vi "V2analysis.vi"(0 "node_in":T2, 1 "VIPathMap":map{string, bool}(c390), 2 "GObj引用句柄":refnum<vi>, 3 "additional_params":T1, 4 "集合":set{string}(c389)) -> (7 "node_out":T2, 8 "VIPathMap 2":map{string, bool}(c390), 10 "集合 2":set{string}(c389))   [LabVIEW 2020]
uses:
  node.ctl
  terminalData.ctl
  terminal_type.ctl
  terminal_direction.ctl
  additional_params.ctl
panel:
  out "依赖关系:丢失依赖关系名称":string[](array[string])
  out "result string":string
  # "tunnel/judge/shift?"
  # "tunnel/judge/shift?"
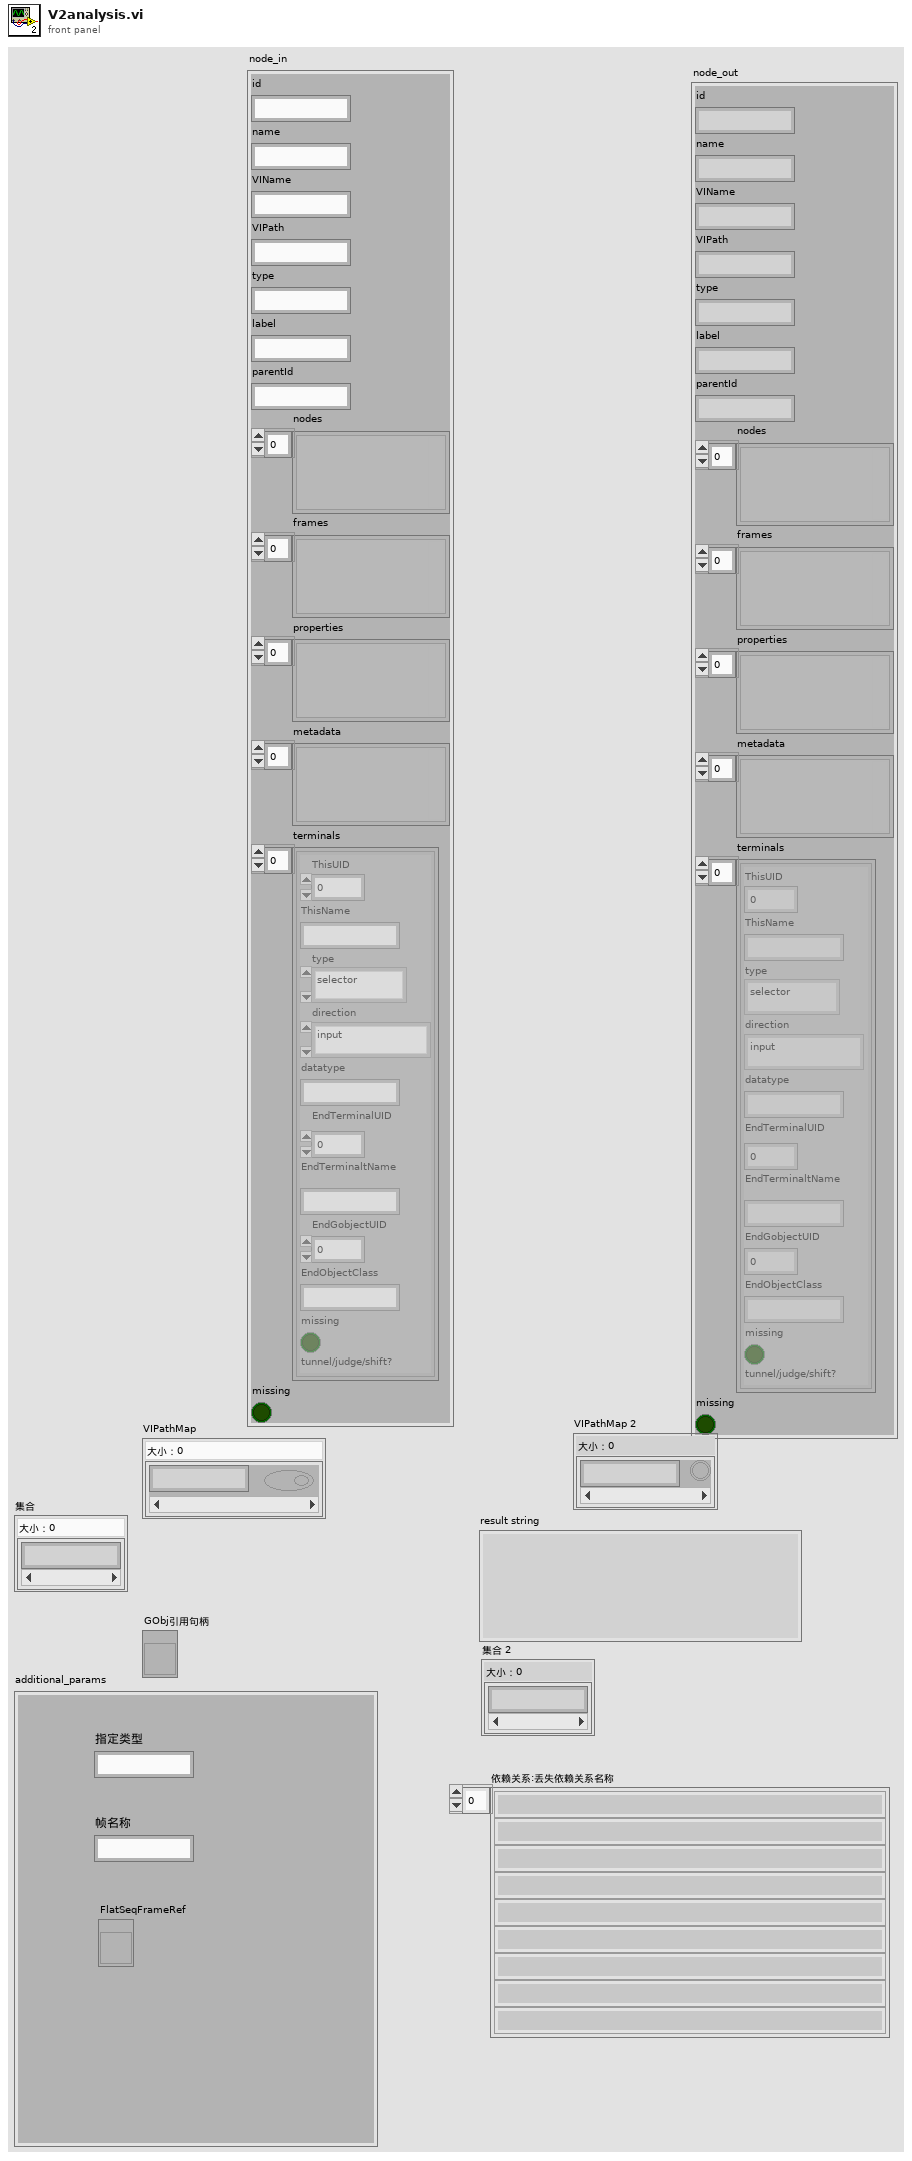
[diagram p1: front panel]
types:
  T1 = typedef "additional_params.ctl" = cluster{"指定类型":string, "帧名称":string, "FlatSeqFrameRef":refnum<vi>}
  T2 = typedef "node.ctl" = cluster{"id":string, "name":string, "VIName":string, "VIPath":string, "type":string, "label":string, "parentId":string, "nodes":variant[], "frames":variant[], "properties":variant[], "metadata":variant[], "terminals":T3[], "missing":bool}
  T3 = typedef "terminalData.ctl" = cluster{"ThisUID":i32, "ThisName":string, "type":T4, "direction":T5, "datatype":string, "EndTerminalUID":i32, "EndTerminaltName":string, "EndGobjectUID":i32, "EndObjectClass":string, "missing":bool}
  T4 = typedef "terminal_type.ctl" = enum16{"selector", "tunnel", "shift", "timeout", "normal", "floating"}
  T5 = typedef "terminal_direction.ctl" = enum16{"input", "output"}
  T6 = cluster{"casename":string, "subdia_text":string}[]
  T7 = cluster{"seq_name":string, "subdia_text":string}[]
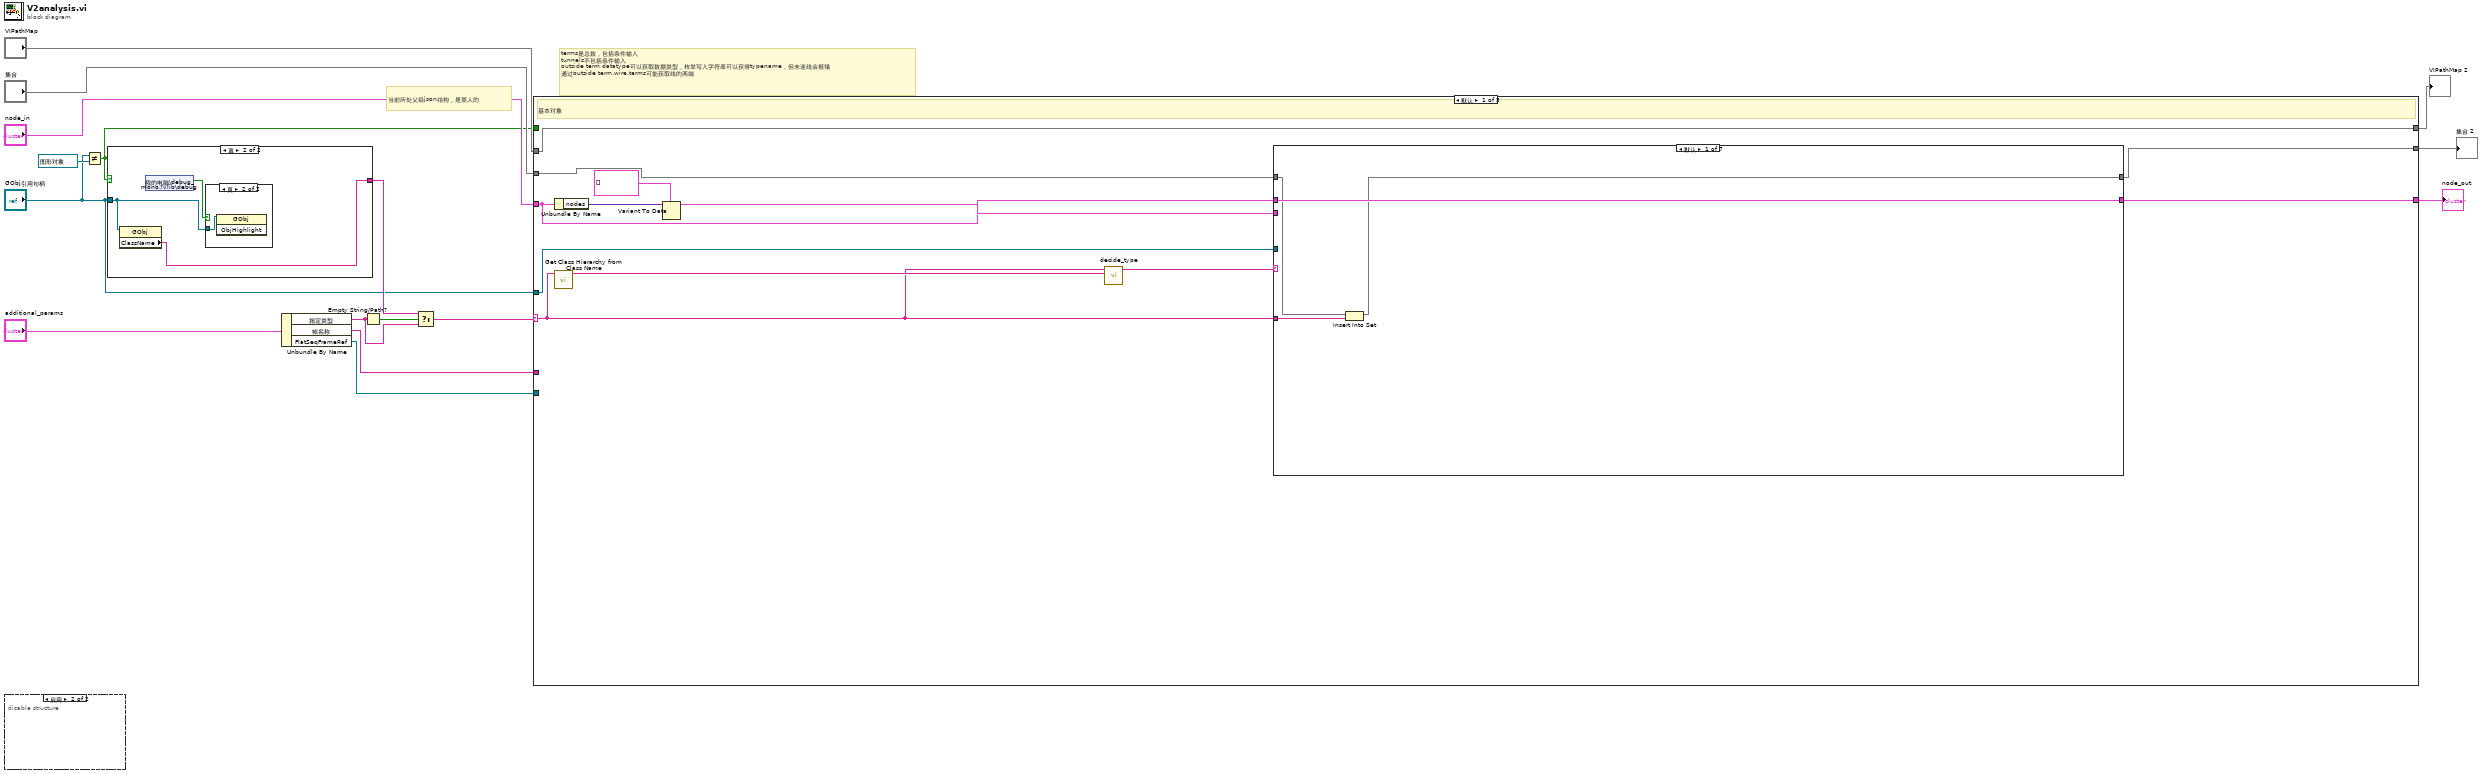
[diagram p0: block diagram]
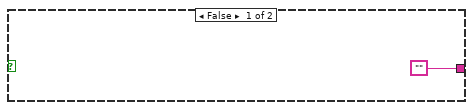
[diagram p2: hidden frame]
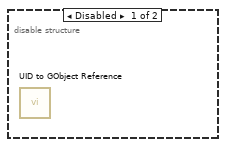
[diagram p4: hidden frame]
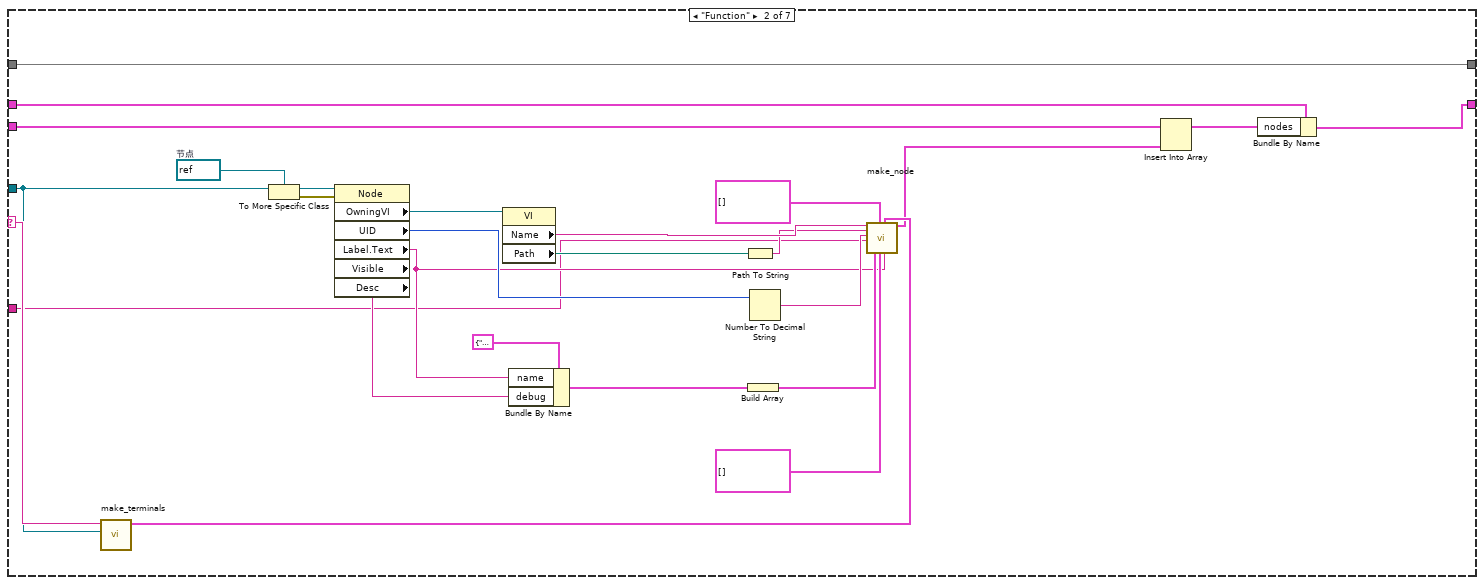
[diagram p5: hidden frame]
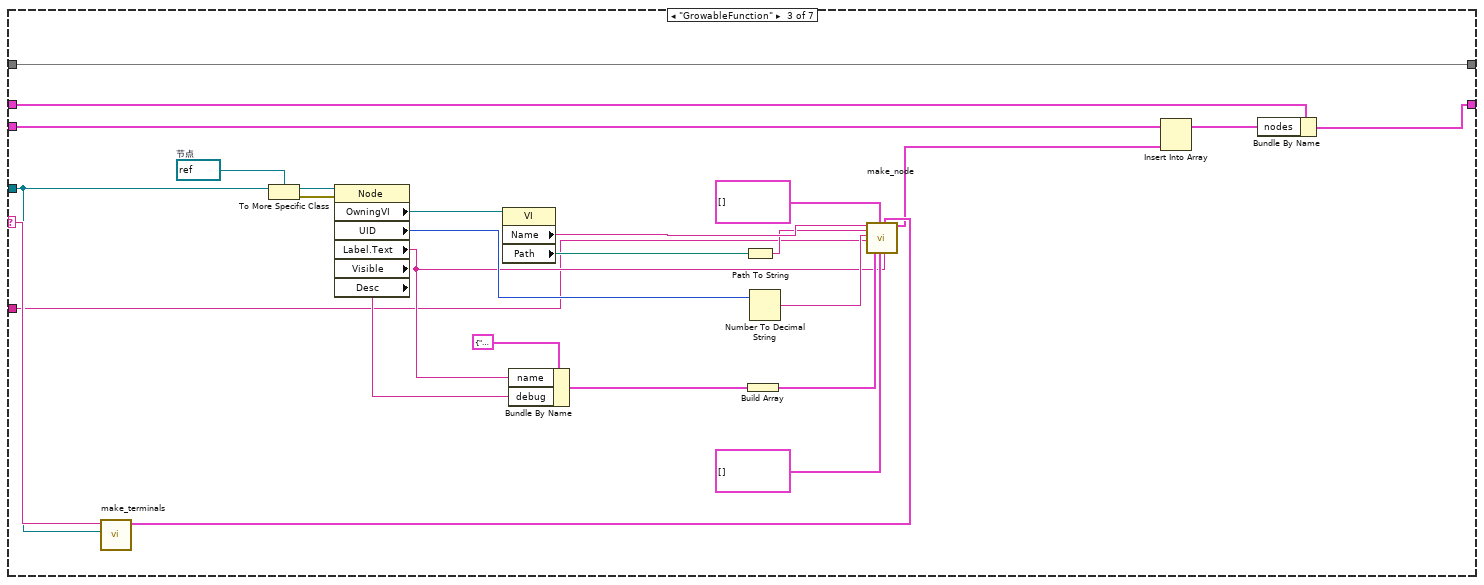
[diagram p6: hidden frame]
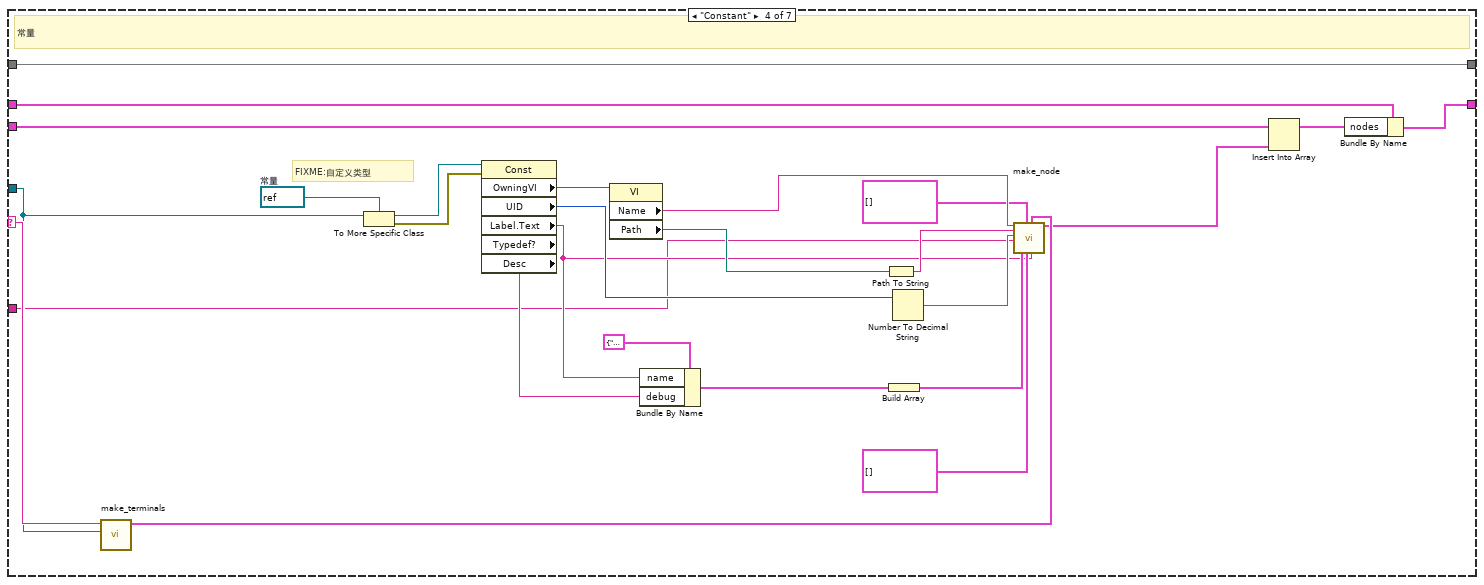
[diagram p7: hidden frame]
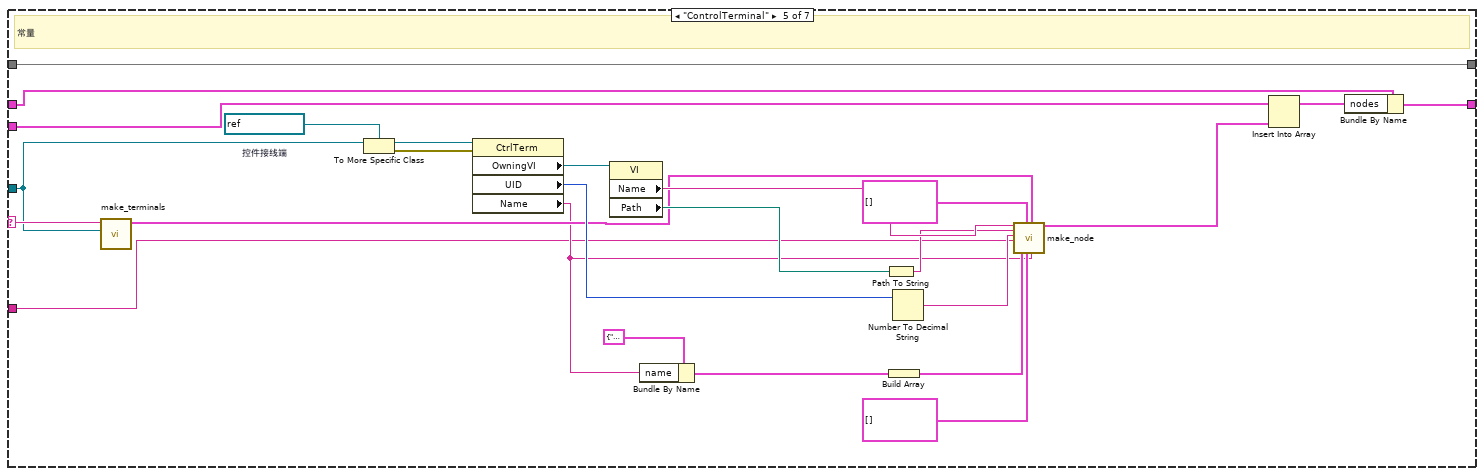
[diagram p8: hidden frame]
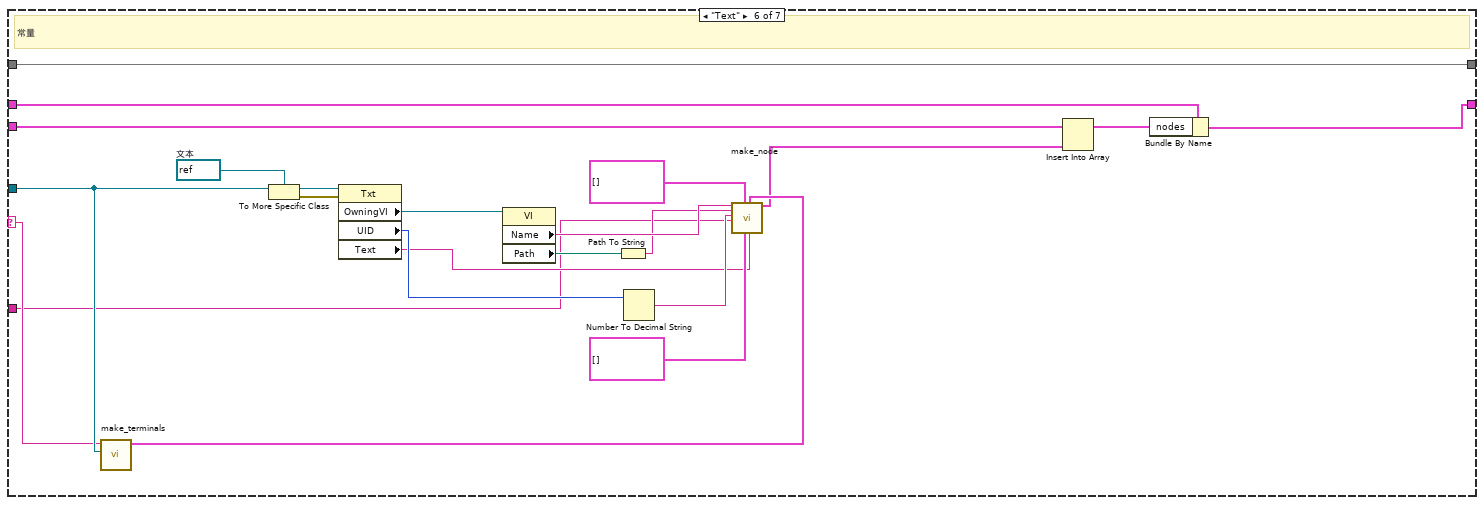
[diagram p9: hidden frame]
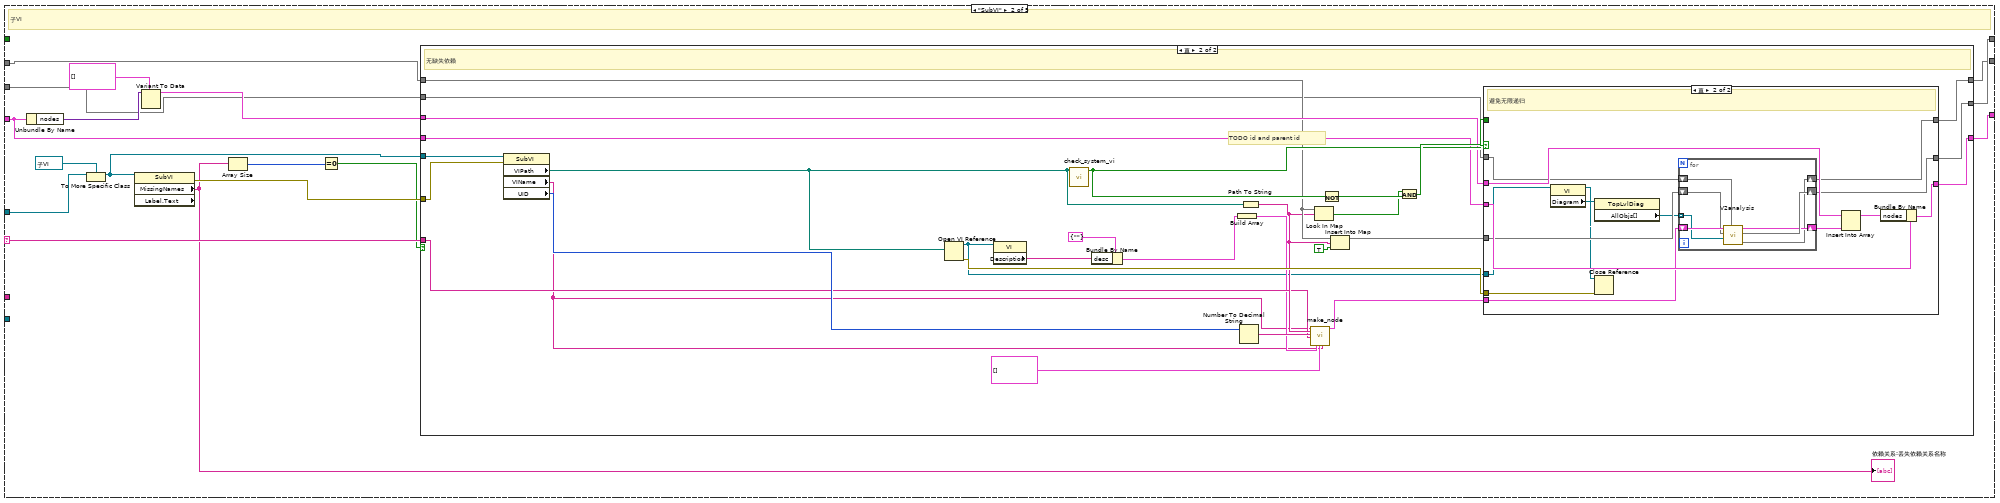
[diagram p11: hidden frame]
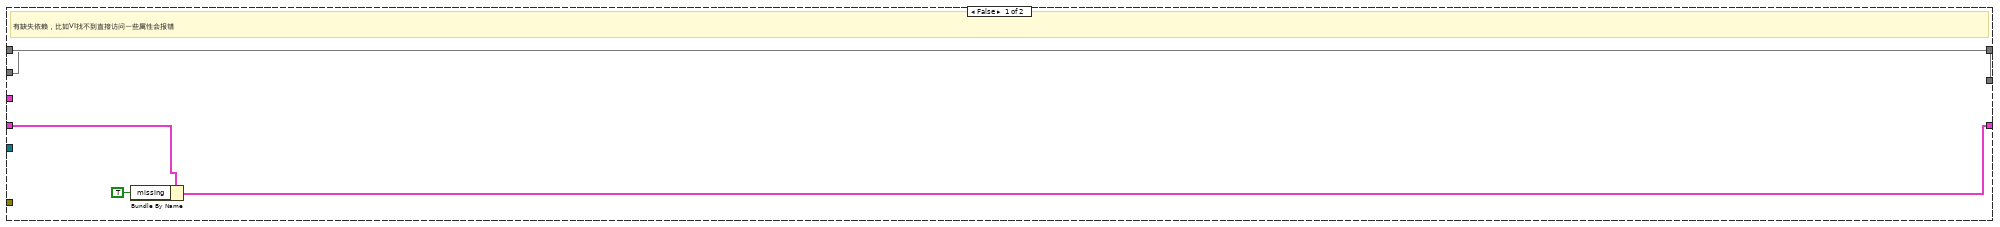
[diagram p12: hidden frame]
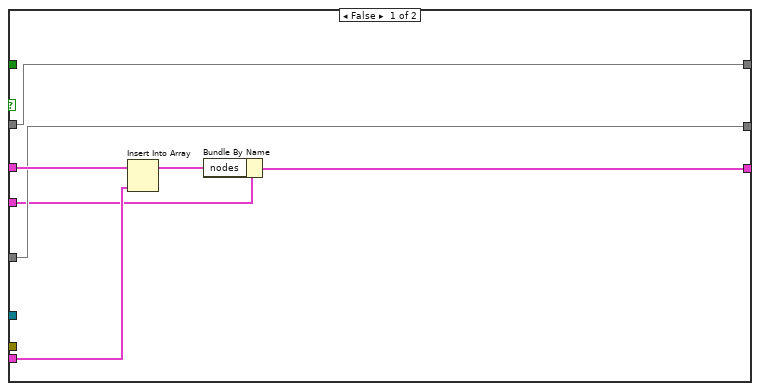
[diagram p13: hidden frame]
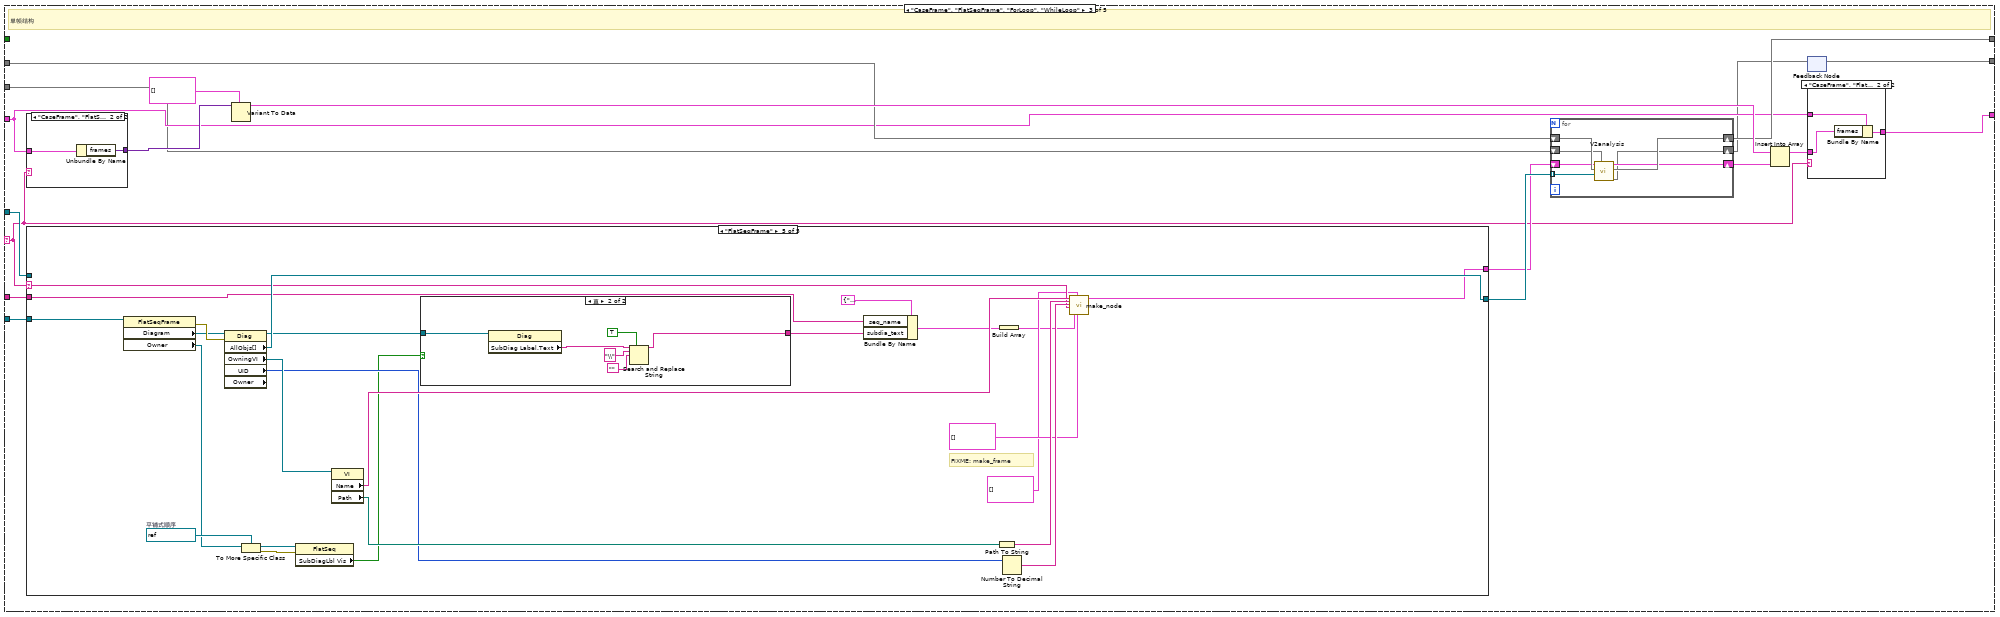
[diagram p14: hidden frame]
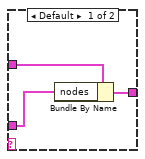
[diagram p15: hidden frame]
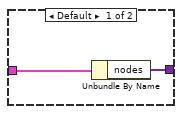
[diagram p16: hidden frame]
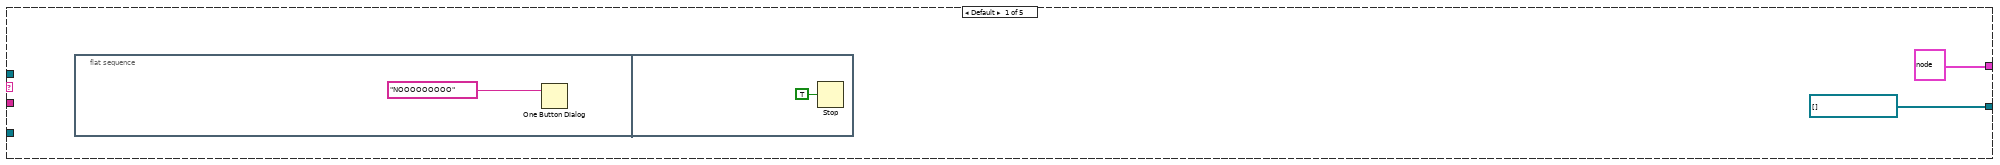
[diagram p17: hidden frame]
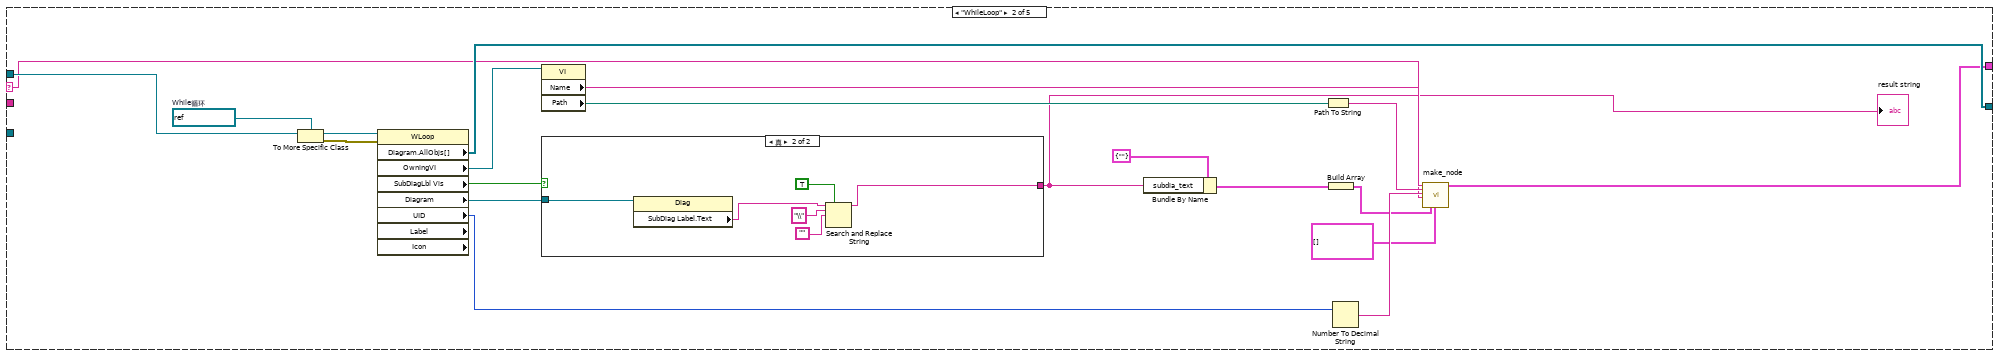
[diagram p18: hidden frame]
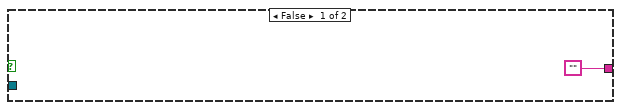
[diagram p19: hidden frame]
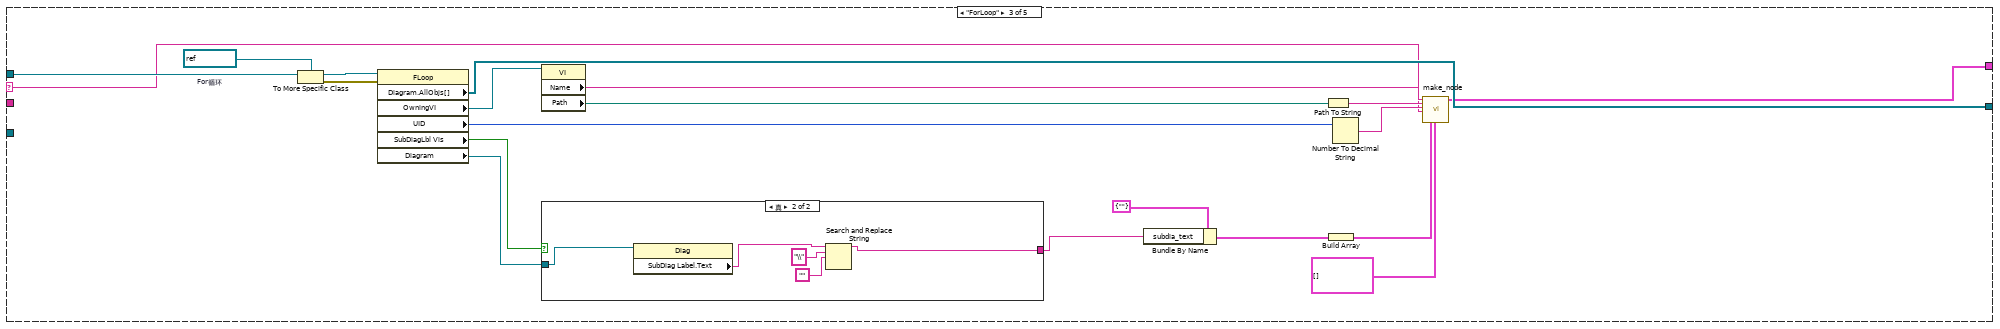
[diagram p20: hidden frame]
diagram:
  # "terms是总数，包括条件输入\ntunnels不包括条件输入\noutside term datatype可以获取数据类型，枚举写入字符串可以获得typename，但未连线会报错\n通过outside term.wire.terms可能获取线的两端"
  # "当前所处父级json结构，是某人的"
  n1 = disable-structure shown="启用" {
    frame Disabled {
      n2 = call <vilib>:"UID to GObject Reference.vi"() -> ()  [unwired: 9 in, 3 out]
    }
    frame Enabled {
    }
  }
  n3 = Not Equal? ("不等于？")(x="GObj引用句柄", y=refnum<vi> refnum ("GObj引用句柄")) -> (x != y?=w1:bool)
  n4 = case shown="真" w1 {
    tunnel: ["" ("空字符串常量") w20] -> w7
    tunnel: "GObj引用句柄" -> [_ w19]
    frame False {
    }
    frame True {
      n5 = property on="属性节点" class="GObj"(reference=w19) -> ("ClassName"=w20:string)  [unwired: 1 in, 2 out]
      n6 = shared-variable "我的电脑\\debug_mono.lvlib\\debug"() -> (w18:bool)  [unwired: 1 in, 1 out]
      n7 = case shown="真" w18 {
        tunnel: w19 -> [_ w21]
        frame False {
        }
        frame True {
          n8 = invoke on="调用节点" class="GObj" method="ObjHighlight"(reference=w21) -> ()  [unwired: 2 in, 3 out]
        }
      }
    }
  }
  n9 = Unbundle By Name ("按名称解除捆绑")("additional_params") -> ("指定类型"=w9:string, "帧名称"=w8:string, "FlatSeqFrameRef"=w4:refnum<vi>)
  n10 = Empty String/Path? ("空字符串/路径？")(string/path=w9) -> (empty?=w12:bool)
  n11 = Select ("选择")(t=w7, s=w12, f=w9) -> (s? t:f=w11:string)
  n12 = case shown="默认" w11 {
    selector: w11 -> [w22 w172 w252 w417 w521]
    tunnel: "GObj引用句柄" -> [w25 w179 w262 w418 w494]
    tunnel: [w28 w181 w250 w410 w514] -> w15
    tunnel: "node_in" -> [w29 w176 w253 w412 w516]
    tunnel: "VIPathMap" -> [w33 w174 w254 w408 w512]
    tunnel: [w33 w173 w257 w409 w513] -> w13
    tunnel: w8 -> [_ _ w249 _ _]
    tunnel: "集合" -> [w24 w171 w246 w403 w508]
    tunnel: [w23 w170 w247 w402 w507] -> w5
    tunnel: w4 -> [_ _ w245 _ _]
    tunnel: w1 -> [_ _ _ _ _]
    frame Default {
      # "基本对象"
      n13 = Unbundle By Name ("按名称解除捆绑")(w29) -> ("nodes"=w32:variant[])
      n14 = call <vilib>:"Get Class Hierarchy from Class Name.vi"("Class Name"=w22) -> ("Class Hierarchy"=w27:string[])  [unwired: 9 in, 1 out]
      n15 = Variant To Data ("变体至数据转换")(type=T2[] [], Variant=w32) -> (data=w30:T2[])  [unwired: 1 in, 1 out]
      n16 = call "decide_type.vi"("Class Hierarchy"=w27, "OriginalClassname"=w22) -> ("OutputType"=w26:string)  [unwired: 9 in]
      n17 = case shown="默认" w26 {
        selector: w26 -> [_ w52 w78 w104 w129 w142 _]
        tunnel: w25 -> [_ w43 w69 w95 w120 w146 _]
        tunnel: w30 -> [_ w48 w74 w100 w125 w151 _]
        tunnel: w29 -> [w37 w46 w72 w98 w123 w149 w164]
        tunnel: [w37 w44 w70 w96 w121 w147 w164] -> w28
        tunnel: w24 -> [w36 w39 w65 w91 w117 w143 w163]
        tunnel: [w35 w39 w65 w91 w117 w143 w163] -> w23
        tunnel: w22 -> [w34 w38 w64 w90 w116 w141 _]
        frame Default {
          n18 = Insert Into Set ("插入集合")(10:w34, 11:w36) -> (3:w35:set{string})  [unwired: 1 out]
        }
        frame "Function" {
          w61 = refnum<vi> refnum  # 节点
          n19 = call "make_terminals.vi"("GObj引用句柄"=w43, "node_type"=w52) -> ("terminals_out"=w53:T3[])  [unwired: 9 in]
          n20 = To More Specific Class ("转换为特定的类")(target class=w61, reference=w43) -> (specific class reference=w63:refnum<vi>, error out=w62:errorcluster)  [unwired: 1 in]
          n21 = property on="属性节点" class="Node" props=["OwningVI", "UID", "Label", "Text", "Visible", "Desc"](reference=w63, error in=w62) -> ("OwningVI"=w60:refnum<vi>, "UID"=w57:i32, "Label.Text"=w40:string, "Desc"=w41:string)  [unwired: 3 out]
          n22 = property on="属性节点" class="VI"(reference=w60) -> ("Name"=w59:string, "Path"=w58:path)  [unwired: 1 in, 2 out]
          n23 = Bundle By Name ("按名称捆绑")(cluster=cluster{"name":string, "debug":string} {"name"="", "debug"=""}, "name"=w40, "debug"=w41) -> (w50:cluster{"name":string, "debug":string})
          n24 = Path To String ("路径至字符串转换")(path=w58) -> (string=w42:string)
          n25 = Build Array ("创建数组")(w50) -> (w49:cluster{"name":string, "debug":string}[])
          n26 = Number To Decimal String ("数值至十进制数字符串转换")(number=w57) -> (decimal integer string=w56:string)  [unwired: 1 in]
          n27 = call "make_node.vi"("VIName"=w59, "VIPath"=w42, "id"=w56, "type"=w38, "metadata"=w49, "frames"=T2[] [] ("nodes"), "nodes"=T2[] [], "terminals"=w53, "name"=w40) -> ("node"=w47:T2)  [unwired: 10 in]
          n28 = Insert Into Array ("数组插入")(array=w48, new element=w47) -> (w45:T2[])  [unwired: 1 in]
          n29 = Bundle By Name ("按名称捆绑")(cluster=w46, "nodes"=w45) -> (w44:T2)
        }
        frame "GrowableFunction" {
          w87 = refnum<vi> refnum  # 节点
          n30 = call "make_terminals.vi"("GObj引用句柄"=w69, "node_type"=w78) -> ("terminals_out"=w79:T3[])  [unwired: 9 in]
          n31 = To More Specific Class ("转换为特定的类")(target class=w87, reference=w69) -> (specific class reference=w89:refnum<vi>, error out=w88:errorcluster)  [unwired: 1 in]
          n32 = property on="属性节点" class="Node" props=["OwningVI", "UID", "Label", "Text", "Visible", "Desc"](reference=w89, error in=w88) -> ("OwningVI"=w86:refnum<vi>, "UID"=w83:i32, "Label.Text"=w66:string, "Desc"=w67:string)  [unwired: 3 out]
          n33 = property on="属性节点" class="VI"(reference=w86) -> ("Name"=w85:string, "Path"=w84:path)  [unwired: 1 in, 2 out]
          n34 = Bundle By Name ("按名称捆绑")(cluster=cluster{"name":string, "debug":string} {"name"="", "debug"=""}, "name"=w66, "debug"=w67) -> (w76:cluster{"name":string, "debug":string})
          n35 = Path To String ("路径至字符串转换")(path=w84) -> (string=w68:string)
          n36 = Build Array ("创建数组")(w76) -> (w75:cluster{"name":string, "debug":string}[])
          n37 = Number To Decimal String ("数值至十进制数字符串转换")(number=w83) -> (decimal integer string=w82:string)  [unwired: 1 in]
          n38 = call "make_node.vi"("VIName"=w85, "VIPath"=w68, "id"=w82, "type"=w64, "metadata"=w75, "frames"=T2[] [] ("nodes"), "nodes"=T2[] [], "terminals"=w79, "name"=w66) -> ("node"=w73:T2)  [unwired: 10 in]
          n39 = Insert Into Array ("数组插入")(array=w74, new element=w73) -> (w71:T2[])  [unwired: 1 in]
          n40 = Bundle By Name ("按名称捆绑")(cluster=w72, "nodes"=w71) -> (w70:T2)
        }
        frame "Constant" {
          w113 = refnum<vi> refnum  # 常量
          # "FIXME:自定义类型"
          # "常量"
          n41 = call "make_terminals.vi"("GObj引用句柄"=w95, "node_type"=w104) -> ("terminals_out"=w105:T3[])  [unwired: 9 in]
          n42 = To More Specific Class ("转换为特定的类")(target class=w113, reference=w95) -> (specific class reference=w115:refnum<vi>, error out=w114:errorcluster)  [unwired: 1 in]
          n43 = property on="属性节点" class="Const" props=["OwningVI", "UID", "Label", "Text", "Typedef?", "Desc"](reference=w115, error in=w114) -> ("OwningVI"=w112:refnum<vi>, "UID"=w109:i32, "Label.Text"=w92:string, "Desc"=w93:string)  [unwired: 3 out]
          n44 = property on="属性节点" class="VI"(reference=w112) -> ("Name"=w111:string, "Path"=w110:path)  [unwired: 1 in, 2 out]
          n45 = Bundle By Name ("按名称捆绑")(cluster=cluster{"name":string, "debug":string} {"name"="", "debug"=""}, "name"=w92, "debug"=w93) -> (w102:cluster{"name":string, "debug":string})
          n46 = Path To String ("路径至字符串转换")(path=w110) -> (string=w94:string)
          n47 = Build Array ("创建数组")(w102) -> (w101:cluster{"name":string, "debug":string}[])
          n48 = Number To Decimal String ("数值至十进制数字符串转换")(number=w109) -> (decimal integer string=w108:string)  [unwired: 1 in]
          n49 = call "make_node.vi"("VIName"=w111, "VIPath"=w94, "id"=w108, "type"=w90, "metadata"=w101, "frames"=T2[] [] ("nodes"), "nodes"=T2[] [], "terminals"=w105, "name"=w92) -> ("node"=w99:T2)  [unwired: 10 in]
          n50 = Insert Into Array ("数组插入")(array=w100, new element=w99) -> (w97:T2[])  [unwired: 1 in]
          n51 = Bundle By Name ("按名称捆绑")(cluster=w98, "nodes"=w97) -> (w96:T2)
        }
        frame "ControlTerminal" {
          w138 = refnum<vi> refnum  # 控件接线端
          # "常量"
          n52 = call "make_terminals.vi"("GObj引用句柄"=w120, "node_type"=w129) -> ("terminals_out"=w130:T3[])  [unwired: 9 in]
          n53 = To More Specific Class ("转换为特定的类")(target class=w138, reference=w120) -> (specific class reference=w140:refnum<vi>, error out=w139:errorcluster)  [unwired: 1 in]
          n54 = property on="属性节点" class="CtrlTerm"(reference=w140, error in=w139) -> ("OwningVI"=w137:refnum<vi>, "UID"=w134:i32, "Name"=w118:string)  [unwired: 2 out]
          n55 = property on="属性节点" class="VI"(reference=w137) -> ("Name"=w136:string, "Path"=w135:path)  [unwired: 1 in, 2 out]
          n56 = Bundle By Name ("按名称捆绑")(cluster=cluster{"name":string, "debug":string} {"name"="", "debug"=""}, "name"=w118) -> (w127:cluster{"name":string, "debug":string})
          n57 = Path To String ("路径至字符串转换")(path=w135) -> (string=w119:string)
          n58 = Build Array ("创建数组")(w127) -> (w126:cluster{"name":string, "debug":string}[])
          n59 = Number To Decimal String ("数值至十进制数字符串转换")(number=w134) -> (decimal integer string=w133:string)  [unwired: 1 in]
          n60 = call "make_node.vi"("VIName"=w136, "VIPath"=w119, "id"=w133, "type"=w116, "metadata"=w126, "frames"=T2[] [] ("nodes"), "nodes"=T2[] [], "terminals"=w130, "name"=w118) -> ("node"=w124:T2)  [unwired: 10 in]
          n61 = Insert Into Array ("数组插入")(array=w125, new element=w124) -> (w122:T2[])  [unwired: 1 in]
          n62 = Bundle By Name ("按名称捆绑")(cluster=w123, "nodes"=w122) -> (w121:T2)
        }
        frame "Text" {
          w160 = refnum<vi> refnum  # 文本
          # "常量"
          n63 = call "make_terminals.vi"("GObj引用句柄"=w146, "node_type"=w142) -> ("terminals_out"=w152:T3[])  [unwired: 9 in]
          n64 = To More Specific Class ("转换为特定的类")(target class=w160, reference=w146) -> (specific class reference=w162:refnum<vi>, error out=w161:errorcluster)  [unwired: 1 in]
          n65 = property on="属性节点" class="Txt"(reference=w162, error in=w161) -> ("OwningVI"=w159:refnum<vi>, "UID"=w156:i32, "Text"=w144:string)  [unwired: 2 out]
          n66 = property on="属性节点" class="VI"(reference=w159) -> ("Name"=w158:string, "Path"=w157:path)  [unwired: 1 in, 2 out]
          n67 = Path To String ("路径至字符串转换")(path=w157) -> (string=w145:string)
          n68 = Number To Decimal String ("数值至十进制数字符串转换")(number=w156) -> (decimal integer string=w155:string)  [unwired: 1 in]
          n69 = call "make_node.vi"("VIName"=w158, "VIPath"=w145, "id"=w155, "type"=w141, "frames"=T2[] [] ("nodes"), "nodes"=T2[] [], "terminals"=w152, "name"=w144) -> ("node"=w150:T2)  [unwired: 11 in]
          n70 = Insert Into Array ("数组插入")(array=w151, new element=w150) -> (w148:T2[])  [unwired: 1 in]
          n71 = Bundle By Name ("按名称捆绑")(cluster=w149, "nodes"=w148) -> (w147:T2)
        }
        frame "Decoration" {
        }
      }
    }
    frame "SubVI" {
      # "子VI"
      n72 = Unbundle By Name ("按名称解除捆绑")(w176) -> ("nodes"=w178:variant[])
      n73 = To More Specific Class ("转换为特定的类")(target class=refnum<vi> refnum ("引用"), reference=w179) -> (specific class reference=w168:refnum<vi>)  [unwired: 1 in, 1 out]
      n74 = property on="属性节点" class="SubVI" props=["MissingNames", "Label", "Text"](reference=w168) -> (error out=w169:errorcluster, "MissingNames"=w167:string[])  [unwired: 1 in, 2 out]
      "依赖关系:丢失依赖关系名称" <- w167
      n75 = Variant To Data ("变体至数据转换")(type=T2[] [], Variant=w178) -> (data=w175:T2[])  [unwired: 1 in, 1 out]
      n76 = Array Size(array=w167) -> (size(s)=w166:i32)
      n77 = Equal To 0?(x=w166) -> (x = 0?=w165:bool)
      n78 = case shown="真" w165 {
        tunnel: [w182 w215] -> w181
        tunnel: w176 -> [w184 w210]
        tunnel: w175 -> [_ w209]
        tunnel: w174 -> [w186 w207]
        tunnel: [w186 w205] -> w173
        tunnel: w172 -> [_ w201]
        tunnel: w171 -> [w185 w190]
        tunnel: [w185 w189] -> w170
        tunnel: w169 -> [_ w188]
        tunnel: w168 -> [_ w187]
        frame False {
          # "有缺失依赖，比如VI找不到直接访问一些属性会报错"
          n79 = Bundle By Name(cluster=w184, "missing"=TRUE) -> (w182:T2)
        }
        frame True {
          # "TODO id and parent id"
          # "无缺失依赖"
          n80 = property on="属性节点" class="SubVI"(reference=w187, error in=w188) -> ("VIPath"=w192:path, "VIName"=w191:string, "UID"=w203:i32)  [unwired: 2 out]
          n81 = Open VI Reference ("打开VI引用")(vi path=w192) -> (vi reference=w194:refnum<vi>, error out=w212:errorcluster)  [unwired: 5 in]
          n82 = property on="属性节点" class="VI"(reference=w194) -> ("Description"=w193:string)  [unwired: 1 in, 2 out]
          n83 = call "check_system_vi.vi"("VIPath"=w192) -> ("布尔 2"=w211:bool)  [unwired: 9 in, 1 out]
          n84 = Bundle By Name ("按名称捆绑")(cluster=cluster{"desc":string} {"desc"=""}, "desc"=w193) -> (w196:cluster{"desc":string})
          n85 = Build Array ("创建数组")(w196) -> (w195:cluster{"desc":string}[])
          n86 = Number To Decimal String ("数值至十进制数字符串转换")(number=w203) -> (decimal integer string=w202:string)  [unwired: 1 in]
          n87 = Path To String ("路径至字符串转换")(path=w192) -> (string=w204:string)
          n88 = call "make_node.vi"("VIName"=w191, "VIPath"=w204, "id"=w202, "type"=w201, "metadata"=w195, "nodes"=T2[] [], "name"=w191) -> ("node"=w199:T2)  [unwired: 12 in]
          n89 = Look In Map ("在映射表中查找")(map=w207, key=w204) -> (key not found?=w208:bool)  [unwired: 1 in, 1 out]
          n90 = Not ("非")(x=w211) -> (.not. x?=w213:bool)
          n91 = Insert Into Map ("插入映射表")(map in=w207, key=w204, value=TRUE ("值")) -> (map out=w206:map{string, bool})  [unwired: 2 out]
          n92 = And ("与")(x=w208, y=w213) -> (x .and. y?=w214:bool)
          n93 = case shown="真" w214 {
            tunnel: w210 -> [w218 w236]
            tunnel: w209 -> [w221 w237]
            tunnel: [w217 w234] -> w215
            tunnel: w212 -> [_ w226]
            tunnel: w211 -> [_ _]
            tunnel: w206 -> [w219 w233]
            tunnel: [w219 w232] -> w205
            tunnel: w199 -> [w220 w230]
            tunnel: w194 -> [_ w228]
            tunnel: w190 -> [w216 w224]
            tunnel: [w216 w223] -> w189
            frame False {
              n94 = Insert Into Array ("数组插入")(array=w221, new element=w220) -> (w222:T2[])  [unwired: 1 in]
              n95 = Bundle By Name ("按名称捆绑")(cluster=w218, "nodes"=w222) -> (w217:T2)
            }
            frame True {
              # "避免无限递归"
              n96 = property on="属性节点" class="VI"(reference=w228) -> (reference out=w225:refnum<vi>, "Diagram"=w227:refnum<vi>)  [unwired: 1 in, 1 out]
              n97 = property on="属性节点" class="TopLvlDiag"(reference=w227) -> ("AllObjs[]"=w229:refnum<vi>[])  [unwired: 1 in, 2 out]
              n98 = Close Reference ("关闭引用")(reference=w225, error in (no error)=w226) -> ()  [unwired: 1 out]
              n99 = for {
                shift-right: [w240] -> w231
                shift-left: w230 -> [w244]
                tunnel: w229 -> [w242] mode=indexing
                shift-right: [w241] -> w232
                shift-left: w233 -> [w243]
                shift-right: [w238] -> w223
                shift-left: w224 -> [w239]
                n100 = call "V2analysis.vi"("node_in"=w244, "VIPathMap"=w243, "GObj引用句柄"=w242, "集合"=w239) -> ("node_out"=w240:T2, "VIPathMap 2"=w241:map{string, bool}, "集合 2"=w238:set{string})  [unwired: 4 in]
              }
              n101 = Insert Into Array ("数组插入")(array=w237, new element=w231) -> (w235:T2[])  [unwired: 1 in]
              n102 = Bundle By Name ("按名称捆绑")(cluster=w236, "nodes"=w235) -> (w234:T2)
            }
          }
        }
      }
    }
    frame "CaseFrame", "FlatSeqFrame", "ForLoop", "WhileLoop" {
      # "单帧结构"
      n103 = case shown="\"CaseFrame\", \"FlatSeqFrame\"" w252 {
        tunnel: [w270 w272] -> w260
        tunnel: w253 -> [w269 w271]
        frame Default {
          n104 = Unbundle By Name ("按名称解除捆绑")(w269) -> ("nodes"=w270:variant[])
        }
        frame "CaseFrame", "FlatSeqFrame" {
          n105 = Unbundle By Name ("按名称解除捆绑")(w271) -> ("frames"=w272:variant[])
        }
      }
      n106 = case "条件结构" shown="\"FlatSeqFrame\"" w252 {
        selector: w252 -> [_ w290 w318 w352 w387]
        tunnel: w262 -> [_ w303 w327 w360 _]
        tunnel: [refnum<vi>[] [] ("Diagram.AllObjs[]") w299 w326 w359 w394] -> w256
        tunnel: [T2 {"id"="", "name"="", "VIName"="", "VIPath"="", "type"="", "label"="", "parentId"="", "nodes"=[], "frames"=[], "properties"=[], "metadata"=[], "terminals"=[], "missing"=FALSE} ("node") w288 w316 w350 w385] -> w255
        tunnel: w249 -> [_ _ _ w338 w375]
        tunnel: w245 -> [_ _ _ _ w373]
        frame Default {
          n107 = flat-sequence {
            frame #0 {
              n108 = One Button Dialog ("单按钮对话框")(message="NOOOOOOOOO" ("消息")) -> ()  [unwired: 1 in, 1 out]
            }
            frame #1 {
              n109 = Stop ("停止")(stop? (T)=TRUE ("停止？(T)")) -> ()
            }
          }
        }
        frame "WhileLoop" {
          w300 = refnum<vi> refnum  # While循环
          n110 = To More Specific Class ("转换为特定的类")(target class=w300, reference=w303) -> (specific class reference=w302:refnum<vi>, error out=w301:errorcluster)  [unwired: 1 in]
          n111 = property on="属性节点" class="WLoop" props=["Diagram", "AllObjs[]", "OwningVI", "SubDiagLbl Vis", "Diagram", "UID", "Label", "Icon"](reference=w302, error in=w301) -> ("Diagram.AllObjs[]"=w299:refnum<vi>[], "OwningVI"=w298:refnum<vi>, "SubDiagLbl Vis"=w297:bool, "Diagram"=w296:refnum<vi>, "UID"=w292:i32)  [unwired: 4 out]
          n112 = property on="属性节点" class="VI"(reference=w298) -> ("Name"=w295:string, "Path"=w294:path)  [unwired: 1 in, 2 out]
          n113 = case shown="真" w297 {
            tunnel: ["" ("SubDiag Label.Text") w306] -> w286
            tunnel: w296 -> [_ w310]
            frame False {
            }
            frame True {
              n114 = property on="属性节点" class="Diag"(reference=w310) -> ("SubDiag Label.Text"=w307:string)  [unwired: 1 in, 2 out]
              n115 = Search and Replace String ("搜索替换字符串")(replace all?=TRUE ("替换全部？(F)"), input string=w307, search string="\\" ("搜索字符串"), replace string="" ("空字符串常量")) -> (result string=w306:string)  [unwired: 4 in, 3 out]
            }
          }
          "result string" <- w286
          n116 = Bundle By Name ("按名称捆绑")(cluster=cluster{"subdia_text":string} {"subdia_text"=""} ("输入簇"), "subdia_text"=w286) -> (w285:cluster{"subdia_text":string})
          n117 = Path To String ("路径至字符串转换")(path=w294) -> (string=w293:string)
          n118 = Build Array ("创建数组")(w285) -> (w284:cluster{"subdia_text":string}[])
          n119 = Number To Decimal String ("数值至十进制数字符串转换")(number=w292) -> (decimal integer string=w291:string)  [unwired: 1 in]
          n120 = call "make_node.vi"("VIName"=w295, "VIPath"=w293, "id"=w291, "type"=w290, "metadata"=w284, "nodes"=T2[] []) -> ("node"=w288:T2)  [unwired: 13 in]
        }
        frame "ForLoop" {
          w328 = refnum<vi> refnum  # For循环
          n121 = To More Specific Class ("转换为特定的类")(target class=w328, reference=w327) -> (specific class reference=w330:refnum<vi>, error out=w329:errorcluster)  [unwired: 1 in]
          n122 = property on="属性节点" class="FLoop"(reference=w330, error in=w329) -> ("Diagram.AllObjs[]"=w326:refnum<vi>[], "OwningVI"=w325:refnum<vi>, "UID"=w320:i32, "SubDiagLbl Vis"=w311:bool, "Diagram"=w324:refnum<vi>)  [unwired: 2 out]
          n123 = property on="属性节点" class="VI"(reference=w325) -> ("Name"=w323:string, "Path"=w322:path)  [unwired: 1 in, 2 out]
          n124 = case shown="真" w311 {
            tunnel: w324 -> [_ w336]
            tunnel: ["" ("SubDiag Label.Text") w332] -> w313
            frame False {
            }
            frame True {
              n125 = property on="属性节点" class="Diag"(reference=w336) -> ("SubDiag Label.Text"=w335:string)  [unwired: 1 in, 2 out]
              n126 = Search and Replace String ("搜索替换字符串")(input string=w335, search string="\\" ("搜索字符串"), replace string="" ("空字符串常量")) -> (result string=w332:string)  [unwired: 5 in, 3 out]
            }
          }
          n127 = Bundle By Name ("按名称捆绑")(cluster=cluster{"subdia_text":string} {"subdia_text"=""} ("输入簇"), "subdia_text"=w313) -> (w314:cluster{"subdia_text":string})
          n128 = Path To String ("路径至字符串转换")(path=w322) -> (string=w321:string)
          n129 = Build Array ("创建数组")(w314) -> (w312:cluster{"subdia_text":string}[])
          n130 = Number To Decimal String ("数值至十进制数字符串转换")(number=w320) -> (decimal integer string=w319:string)  [unwired: 1 in]
          n131 = call "make_node.vi"("VIName"=w323, "VIPath"=w321, "id"=w319, "type"=w318, "metadata"=w312, "nodes"=T2[] []) -> ("node"=w316:T2)  [unwired: 13 in]
        }
        frame "CaseFrame" {
          w345 = refnum<vi> refnum  # 多帧结构
          w346 = refnum<vi> refnum  # 程序框图
          # "FIXME: make_frame"
          n132 = To More Specific Class ("转换为特定的类")(target class=w346, reference=w360) -> (specific class reference=w362:refnum<vi>, error out=w361:errorcluster)  [unwired: 1 in]
          n133 = property on="属性节点" class="Diag" props=["AllObjs[]", "OwningVI", "UID", "Owner", "Nodes[]"](reference=w362, error in=w361) -> (reference out=w340:refnum<vi>, "AllObjs[]"=w359:refnum<vi>[], "OwningVI"=w358:refnum<vi>, "UID"=w354:i32, "Owner"=w344:refnum<vi>)  [unwired: 2 out]
          n134 = property on="属性节点" class="VI"(reference=w358) -> ("Name"=w357:string, "Path"=w356:path)  [unwired: 1 in, 2 out]
          n135 = To More Specific Class ("转换为特定的类")(target class=w345, reference=w344) -> (specific class reference=w343:refnum<vi>, error out=w342:errorcluster)  [unwired: 1 in]
          n136 = property on="属性节点" class="MFStruct"(reference=w343, error in=w342) -> ("SubDiagLbl Vis"=w341:bool)  [unwired: 2 out]
          n137 = case shown="真" w341 {
            tunnel: ["" ("SubDiag Label.Text") w366] -> w347
            tunnel: w340 -> [_ w365]
            frame False {
            }
            frame True {
              n138 = property on="属性节点" class="Diag"(reference=w365) -> ("SubDiag Label.Text"=w369:string)  [unwired: 1 in, 2 out]
              n139 = Search and Replace String ("搜索替换字符串")(replace all?=TRUE ("替换全部？(F)"), input string=w369, search string="\\" ("搜索字符串"), replace string="" ("空字符串常量")) -> (result string=w366:string)  [unwired: 4 in, 3 out]
            }
          }
          n140 = Bundle By Name ("按名称捆绑")(cluster=cluster{"casename":string, "subdia_text":string} {"casename"="", "subdia_text"=""} ("输入簇"), "casename"=w338, "subdia_text"=w347) -> (w348:cluster{"casename":string, "subdia_text":string})
          n141 = Path To String ("路径至字符串转换")(path=w356) -> (string=w355:string)
          n142 = Build Array ("创建数组")(w348) -> (w337:T6)
          n143 = Number To Decimal String ("数值至十进制数字符串转换")(number=w354) -> (decimal integer string=w353:string)  [unwired: 1 in]
          n144 = call "make_node.vi"("VIName"=w357, "VIPath"=w355, "id"=w353, "type"=w352, "metadata"=w337, "frames"=T2[] [] ("nodes"), "nodes"=T2[] []) -> ("node"=w350:T2)  [unwired: 12 in]
        }
        frame "FlatSeqFrame" {
          w381 = refnum<vi> refnum  # 平铺式顺序
          # "FIXME: make_frame"
          n145 = property on="属性节点" class="FlatSeqFrame"(reference=w373) -> (error out=w372:errorcluster, "Diagram"=w371:refnum<vi>, "Owner"=w370:refnum<vi>)  [unwired: 1 in, 1 out]
          n146 = property on="属性节点" class="Diag" props=["AllObjs[]", "OwningVI", "UID", "Owner"](reference=w371, error in=w372) -> (reference out=w377:refnum<vi>, "AllObjs[]"=w394:refnum<vi>[], "OwningVI"=w393:refnum<vi>, "UID"=w389:i32)  [unwired: 2 out]
          n147 = To More Specific Class ("转换为特定的类")(target class=w381, reference=w370) -> (specific class reference=w380:refnum<vi>, error out=w379:errorcluster)  [unwired: 1 in]
          n148 = property on="属性节点" class="FlatSeq"(reference=w380, error in=w379) -> ("SubDiagLbl Vis"=w378:bool)  [unwired: 2 out]
          n149 = property on="属性节点" class="VI"(reference=w393) -> ("Name"=w392:string, "Path"=w391:path)  [unwired: 1 in, 2 out]
          n150 = case shown="真" w378 {
            tunnel: ["" ("SubDiag Label.Text") w398] -> w382
            tunnel: w377 -> [_ w397]
            frame False {
            }
            frame True {
              n151 = property on="属性节点" class="Diag"(reference=w397) -> ("SubDiag Label.Text"=w401:string)  [unwired: 1 in, 2 out]
              n152 = Search and Replace String ("搜索替换字符串")(replace all?=TRUE ("替换全部？(F)"), input string=w401, search string="\\" ("搜索字符串"), replace string="" ("空字符串常量")) -> (result string=w398:string)  [unwired: 4 in, 3 out]
            }
          }
          n153 = Bundle By Name ("按名称捆绑")(cluster=cluster{"seq_name":string, "subdia_text":string} {"seq_name"="", "subdia_text"=""} ("输入簇"), "seq_name"=w375, "subdia_text"=w382) -> (w383:cluster{"seq_name":string, "subdia_text":string})
          n154 = Path To String ("路径至字符串转换")(path=w391) -> (string=w390:string)
          n155 = Build Array ("创建数组")(w383) -> (w374:T7)
          n156 = Number To Decimal String ("数值至十进制数字符串转换")(number=w389) -> (decimal integer string=w388:string)  [unwired: 1 in]
          n157 = call "make_node.vi"("VIName"=w392, "VIPath"=w390, "id"=w388, "type"=w387, "metadata"=w374, "frames"=T2[] [] ("nodes"), "nodes"=T2[] []) -> ("node"=w385:T2)  [unwired: 12 in]
        }
      }
      n158 = Variant To Data ("变体至数据转换")(type=T2[] [], Variant=w260) -> (data=w258:T2[])  [unwired: 1 in, 1 out]
      n159 = for {
        shift-right: [w277] -> w261
        shift-left: w255 -> [w276]
        shift-right: [w278] -> w257
        shift-left: w254 -> [w279]
        tunnel: w256 -> [w275] mode=indexing
        shift-right: [w273] -> w248
        shift-left: w246 -> [w274]
        n160 = call "V2analysis.vi"("node_in"=w276, "VIPathMap"=w279, "GObj引用句柄"=w275, "集合"=w274) -> ("node_out"=w277:T2, "VIPathMap 2"=w278:map{string, bool}, "集合 2"=w273:set{string})  [unwired: 4 in]
      }
      n161 = Insert Into Array ("数组插入")(array=w258, new element=w261) -> (w251:T2[])  [unwired: 1 in]
      n162 = feedback-in #1(w248) -> ()
      n163 = feedback #1() -> (w247:set{string})  [unwired: 1 in]
      n164 = case shown="\"CaseFrame\", \"FlatSeqFrame\"" w252 {
        tunnel: w253 -> [w265 w268]
        tunnel: w251 -> [w264 w267]
        tunnel: [w263 w266] -> w250
        frame Default {
          n165 = Bundle By Name ("按名称捆绑")(cluster=w265, "nodes"=w264) -> (w263:T2)
        }
        frame "CaseFrame", "FlatSeqFrame" {
          n166 = Bundle By Name ("按名称捆绑")(cluster=w268, "frames"=w267) -> (w266:T2)
        }
      }
    }
    frame "CaseStructure", "DisableStructure", "EventStructure" {
      # "多帧结构"
      n167 = Unbundle By Name ("按名称解除捆绑")(w412) -> ("nodes"=w414:variant[])
      n168 = case shown="\"DisableStructure\"" w417 {
        selector: w417 -> [_ w437 w457 w483]
        tunnel: w418 -> [_ w438 w456 w493]
        tunnel: [T2 {"id"="", "name"="", "VIName"="", "VIPath"="", "type"="", "label"="", "parentId"="", "nodes"=[], "frames"=[], "properties"=[], "metadata"=[], "terminals"=[], "missing"=FALSE} ("node") w444 w462 w481] -> w407
        tunnel: [refnum<vi>[] [] ("Frames[]") w443 w461 w475] -> w406
        tunnel: ["" ("空字符串常量") "CaseFrame" "CaseFrame" "CaseFrame"] -> w405
        tunnel: [string[] [] ("FrameNames") w440 w458 w473] -> w404
        frame "假", Default {
          n169 = flat-sequence {
            frame #0 {
              n170 = One Button Dialog ("单按钮对话框")(message="NOOOOOOOOO" ("消息")) -> ()  [unwired: 1 in, 1 out]
            }
            frame #1 {
              n171 = Stop ("停止")(stop? (T)=TRUE ("停止？(T)")) -> ()
            }
          }
        }
        frame "CaseStructure" {
          w452 = refnum<vi> refnum  # 条件结构
          n172 = call "make_terminals.vi"("GObj引用句柄"=w438, "node_type"=w437) -> ("terminals_out"=w439:T3[])  [unwired: 9 in]
          n173 = To More Specific Class ("转换为特定的类")(target class=w452, reference=w438) -> (specific class reference=w454:refnum<vi>, error out=w453:errorcluster)  [unwired: 1 in]
          n174 = property on="属性节点" class="CaseSel"(reference=w454, error in=w453) -> ("OwningVI"=w451:refnum<vi>, "Frames[]"=w443:refnum<vi>[], "UID"=w447:i32, "FrameNames"=w440:string[])  [unwired: 2 out]
          n175 = property on="属性节点" class="VI"(reference=w451) -> ("Name"=w450:string, "Path"=w449:path)  [unwired: 1 in, 2 out]
          n176 = Path To String ("路径至字符串转换")(path=w449) -> (string=w448:string)
          n177 = Number To Decimal String ("数值至十进制数字符串转换")(number=w447) -> (decimal integer string=w446:string)  [unwired: 1 in]
          n178 = call "make_node.vi"("VIName"=w450, "VIPath"=w448, "id"=w446, "type"=w437, "frames"=T2[] [] ("nodes"), "nodes"=T2[] [], "terminals"=w439) -> ("node"=w444:T2)  [unwired: 12 in]
        }
        frame "EventStructure" {
          w470 = refnum<vi> refnum  # 事件结构
          # "FIXME"
          n179 = call "make_terminals.vi"("GObj引用句柄"=w456, "node_type"=w457) -> ("terminals_out"=w455:T3[])  [unwired: 9 in]
          n180 = To More Specific Class ("转换为特定的类")(target class=w470, reference=w456) -> (specific class reference=w472:refnum<vi>, error out=w471:errorcluster)  [unwired: 1 in]
          n181 = property on="属性节点" class="EvntStruct"(reference=w472, error in=w471) -> ("OwningVI"=w469:refnum<vi>, "Frames[]"=w461:refnum<vi>[], "UID"=w465:i32, "EventSelectors"=w458:string[])  [unwired: 2 out]
          n182 = property on="属性节点" class="VI"(reference=w469) -> ("Name"=w468:string, "Path"=w467:path)  [unwired: 1 in, 2 out]
          n183 = Path To String ("路径至字符串转换")(path=w467) -> (string=w466:string)
          n184 = Number To Decimal String ("数值至十进制数字符串转换")(number=w465) -> (decimal integer string=w464:string)  [unwired: 1 in]
          n185 = call "make_node.vi"("VIName"=w468, "VIPath"=w466, "id"=w464, "type"=w457, "frames"=T2[] [] ("nodes"), "nodes"=T2[] [], "terminals"=w455) -> ("node"=w462:T2)  [unwired: 12 in]
        }
        frame "DisableStructure" {
          w490 = refnum<vi> refnum  # 禁用结构
          # "FIXME"
          # "启用的程序框图帧"
          n186 = To More Specific Class ("转换为特定的类")(target class=w490, reference=w493) -> (specific class reference=w492:refnum<vi>, error out=w491:errorcluster)  [unwired: 1 in]
          n187 = property on="属性节点" class="DisableStructure"(reference=w492, error in=w491) -> ("OwningVI"=w489:refnum<vi>, "Frames[]"=w478:refnum<vi>[], "UID"=w485:i32, "ActiveFrame"=w477:i16)  [unwired: 2 out]
          n188 = property on="属性节点" class="VI"(reference=w489) -> ("Name"=w488:string, "Path"=w487:path)  [unwired: 1 in, 2 out]
          n189 = Index Array ("索引数组")(array=w478, index=w477) -> (element=w476:refnum<vi>)
          n190 = Path To String ("路径至字符串转换")(path=w487) -> (string=w486:string)
          n191 = Build Array ("创建数组")(w476) -> (w475:refnum<vi>[])
          n192 = Number To Decimal String ("数值至十进制数字符串转换")(number=w485) -> (decimal integer string=w484:string)  [unwired: 1 in]
          n193 = call "make_node.vi"("VIName"=w488, "VIPath"=w486, "id"=w484, "type"=w483, "frames"=T2[] [] ("nodes"), "nodes"=T2[] []) -> ("node"=w481:T2)  [unwired: 13 in]
          n194 = Build Array ("创建数组")("启用") -> (w473:string[])
        }
      }
      n195 = Variant To Data ("变体至数据转换")(type=T2[] [], Variant=w414) -> (data=w411:T2[])  [unwired: 1 in, 1 out]
      n196 = for {
        shift-right: [w428] -> w415
        shift-left: w407 -> [w427]
        shift-right: [w429] -> w409
        shift-left: w408 -> [w430]
        tunnel: w406 -> [w426] mode=indexing
        tunnel: w405 -> [w423]
        tunnel: w404 -> [w422] mode=indexing
        shift-right: [w419] -> w402
        shift-left: w403 -> [w420]
        n197 = call "process_frame_text.vi"("字符串"=w422) -> ("result string"=w421:string)  [unwired: 10 in]
        n198 = Bundle By Name ("按名称捆绑")(cluster=T1 {"指定类型"="", "帧名称"="", "FlatSeqFrameRef"=refnum} ("additional_params 2"), "指定类型"=w423, "帧名称"=w421) -> (w424:T1)
        n199 = call "V2analysis.vi"("node_in"=w427, "VIPathMap"=w430, "GObj引用句柄"=w426, "additional_params"=w424, "集合"=w420) -> ("node_out"=w428:T2, "VIPathMap 2"=w429:map{string, bool}, "集合 2"=w419:set{string})  [unwired: 3 in]
      }
      n200 = Insert Into Array ("数组插入")(array=w411, new element=w415) -> (w416:T2[])  [unwired: 1 in]
      n201 = Bundle By Name ("按名称捆绑")(cluster=w412, "nodes"=w416) -> (w410:T2)
    }
    frame "FlatSequence" {
      w504 = refnum<vi> refnum  # 平铺式顺序
      # "多帧结构"
      n202 = Unbundle By Name ("按名称解除捆绑")(w516) -> ("nodes"=w518:variant[])
      n203 = call "make_terminals.vi"("GObj引用句柄"=w494, "node_type"=w521) -> ("terminals_out"=w495:T3[])  [unwired: 9 in]
      n204 = Variant To Data ("变体至数据转换")(type=T2[] [], Variant=w518) -> (data=w515:T2[])  [unwired: 1 in, 1 out]
      n205 = To More Specific Class ("转换为特定的类")(target class=w504, reference=w494) -> (specific class reference=w506:refnum<vi>, error out=w505:errorcluster)  [unwired: 1 in]
      n206 = property on="属性节点" class="FlatSeq"(reference=w506, error in=w505) -> ("OwningVI"=w503:refnum<vi>, "Frames[]"=w510:refnum<vi>[], "UID"=w499:i32)  [unwired: 2 out]
      n207 = property on="属性节点" class="VI"(reference=w503) -> ("Name"=w502:string, "Path"=w501:path)  [unwired: 1 in, 2 out]
      n208 = Path To String ("路径至字符串转换")(path=w501) -> (string=w500:string)
      n209 = Number To Decimal String ("数值至十进制数字符串转换")(number=w499) -> (decimal integer string=w498:string)  [unwired: 1 in]
      n210 = call "make_node.vi"("VIName"=w502, "VIPath"=w500, "id"=w498, "type"=w521, "frames"=T2[] [] ("nodes"), "nodes"=T2[] [], "terminals"=w495) -> ("node"=w511:T2)  [unwired: 12 in]
      n211 = for {
        shift-right: [w530] -> w519
        shift-left: w511 -> [w529]
        shift-right: [w531] -> w513
        shift-left: w512 -> [w532]
        tunnel: w510 -> [w523] mode=indexing
        tunnel: "FlatSeqFrame" -> [w526]
        shift-right: [w524] -> w507
        shift-left: w508 -> [w525]
        n212 = Bundle By Name ("按名称捆绑")(cluster=T1 {"指定类型"="", "帧名称"="", "FlatSeqFrameRef"=refnum} ("additional_params 2"), "指定类型"=w526, "FlatSeqFrameRef"=w523) -> (w527:T1)
        n213 = call "V2analysis.vi"("node_in"=w529, "VIPathMap"=w532, "GObj引用句柄"=refnum<vi> refnum, "additional_params"=w527, "集合"=w525) -> ("node_out"=w530:T2, "VIPathMap 2"=w531:map{string, bool}, "集合 2"=w524:set{string})  [unwired: 3 in]
      }
      n214 = Insert Into Array ("数组插入")(array=w515, new element=w519) -> (w520:T2[])  [unwired: 1 in]
      n215 = Bundle By Name ("按名称捆绑")(cluster=w516, "nodes"=w520) -> (w514:T2)
    }
  }
  "node_out" <- w15
  "VIPathMap 2" <- w13
  "集合 2" <- w5
